vi "Drive Get and use.vi"(0 "Slow Drive":bool, 1 "Y - Axis":dbl, 2 "X - Axis":dbl) -> ()   [LabVIEW 2013]
uses:
  Drive Global.vi
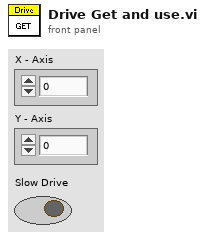
[diagram p1: front panel]
types:
  T1 = cluster{"Axis X":dbl, "Axis Y":dbl, "Slow Drive":bool}
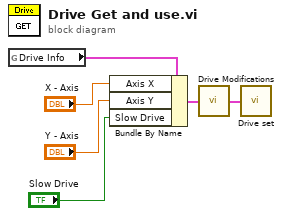
[diagram p0: block diagram]
diagram:
  n1 = global read "Drive Global.vi" "Drive Info"() -> (w6:T1)
  n2 = Bundle By Name(cluster=w6, "Axis X"="X - Axis", "Axis Y"="Y - Axis", "Slow Drive"="Slow Drive") -> (w1:T1)
  n3 = call "Drive Modifications.vi"("Drive Info In"=w1) -> ("Drive Info Out"=w2:T1)
  n4 = call "Drive set.vi"("Drive Info In"=w2) -> ()  [unwired: 1 out]
